vi "Queue Driver LV2.vi"(0 "States":T1[](array[typedef]), 2 "Name":string, 11 "Error In":errorcluster, 13 "Operation":T2=enum."Enqueue") -> (4 "Dequeued State":T1, 15 "error out":errorcluster)   [LabVIEW 2022 SP3, in "Sample PC Template.lvlib"]
doc: "LV2 used for queue operations\nQueue used for enqueue/dequeue of States"
uses:
  Sample PC Template.lvlib
  Typedefs/Data.ctl
  Typedefs/Queue Operations.ctl
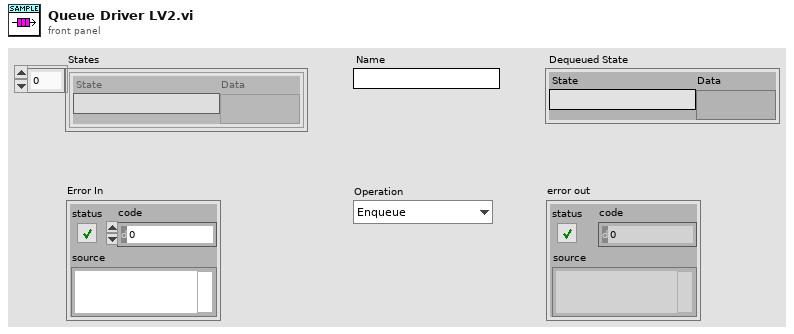
[diagram p1: front panel]
types:
  T1 = typedef "Sample PC Template.lvlib/Data.ctl" = cluster{"State":string, "Data":variant}
  T2 = typedef "Sample PC Template.lvlib/Queue Operations.ctl" = enum16{"Create Q", "Enqueue", "Enstack", "Dequeue", "Flush Q", "Release Q"}
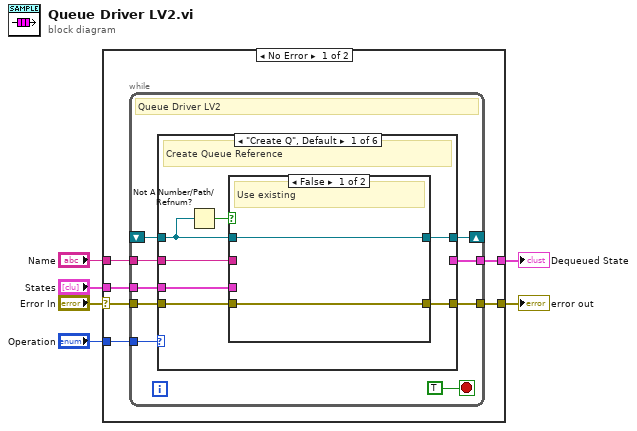
[diagram p0: block diagram]
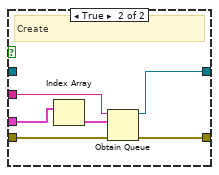
[diagram p2: hidden frame]
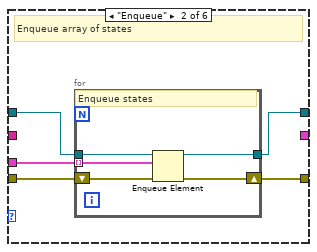
[diagram p3: hidden frame]
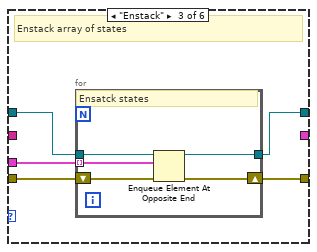
[diagram p4: hidden frame]
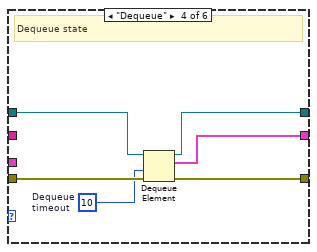
[diagram p5: hidden frame]
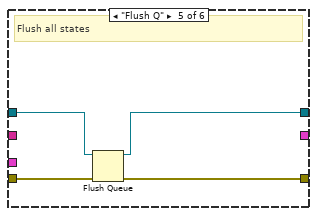
[diagram p6: hidden frame]
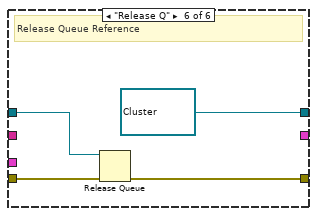
[diagram p7: hidden frame]
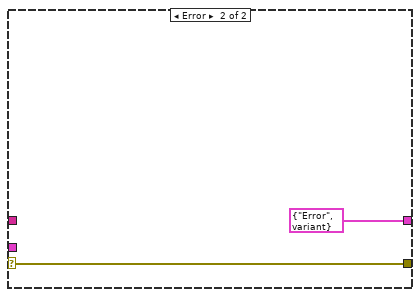
[diagram p8: hidden frame]
diagram:
  n1 = case shown="No Error" "Error In" {
    selector: "Error In" -> [w11 w72]
    tunnel: [w12 w72] -> w5
    tunnel: "Operation" -> [w10 _]
    tunnel: "Name" -> [w9 _]
    tunnel: "States" -> [w8 _]
    tunnel: [w7 T1 {"State"="Error", "Data"=variant} ("Cluster")] -> w1
    frame No Error {
      n2 = while {
        tunnel: [w21] -> w12
        tunnel: w11 -> [w20]
        tunnel: w10 -> [w19]
        tunnel: w9 -> [w16]
        tunnel: w8 -> [w15]
        shift-right: [w17] -> _
        shift-left: _ -> [w18]
        tunnel: [w14] -> w7
        stop <- TRUE stop-if-true
        # "Queue Driver LV2"
        n3 = case shown="\"Create Q\", Default" w19 {
          tunnel: [w27 w41 w51 w62 w66 w70] -> w21
          tunnel: w20 -> [w28 w40 w50 w61 w65 w69]
          tunnel: w18 -> [w22 w39 w49 w60 w64 w68]
          tunnel: [w25 w38 w48 w59 w63 refnum<queue> refnum ("queue out")] -> w17
          tunnel: w16 -> [w26 _ _ _ _ _]
          tunnel: w15 -> [w24 w37 w47 _ _ _]
          tunnel: [_ _ _ w58 _ _] -> w14
          frame "Create Q", Default {
            # "Create Queue Reference"
            n4 = Not A Number/Path/Refnum?(number/path/refnum=w22) -> (NaN/Path/Refnum?=w23:bool)
            n5 = case shown="False" w23 {
              tunnel: w28 -> [w29 w36]
              tunnel: [w29 w35] -> w27
              tunnel: w26 -> [_ w34]
              tunnel: [w30 w33] -> w25
              tunnel: w24 -> [_ w32]
              tunnel: w22 -> [w30 _]
              frame False {
                # "Use existing"
              }
              frame True {
                # "Create"
                n6 = Index Array(array=w32) -> (element=w31:T1)  [unwired: 1 in]
                n7 = Obtain Queue(name (unnamed)=w34, element data type=w31, error in (no error)=w36) -> (queue out=w33:refnum<queue>, error out=w35:errorcluster)  [unwired: 2 in, 1 out]
              }
            }
          }
          frame "Enqueue" {
            # "Enqueue array of states"
            n8 = for {
              tunnel: w39 -> [w44]
              tunnel: [w43] -> w38
              tunnel: w37 -> [w42] mode=indexing
              shift-right: [w46] -> w41
              shift-left: w40 -> [w45]
              # "Enqueue states"
              n9 = Enqueue Element(queue=w44, element=w42, error in (no error)=w45) -> (queue out=w43:refnum<queue>, error out=w46:errorcluster)  [unwired: 1 in, 1 out]
            }
          }
          frame "Enstack" {
            # "Enstack array of states"
            n10 = for {
              tunnel: w49 -> [w54]
              tunnel: [w53] -> w48
              tunnel: w47 -> [w52] mode=indexing
              shift-right: [w56] -> w51
              shift-left: w50 -> [w55]
              # "Ensatck states"
              n11 = Enqueue Element At Opposite End(queue=w54, element=w52, error in (no error)=w55) -> (queue out=w53:refnum<queue>, error out=w56:errorcluster)  [unwired: 1 in, 1 out]
            }
          }
          frame "Dequeue" {
            w57 = 10  # Dequeue timeout
            # "Dequeue state"
            n12 = Dequeue Element(queue=w60, timeout in ms (-1)=w57, error in (no error)=w61) -> (queue out=w59:refnum<queue>, element=w58:T1, error out=w62:errorcluster)  [unwired: 1 out]
          }
          frame "Flush Q" {
            # "Flush all states"
            n13 = Flush Queue(queue=w64, error in (no error)=w65) -> (queue out=w63:refnum<queue>, error out=w66:errorcluster)  [unwired: 1 out]
          }
          frame "Release Q" {
            # "Release Queue Reference"
            n14 = Release Queue(queue=w68, error in (no error)=w69) -> (error out=w70:errorcluster)  [unwired: 1 in, 2 out]
          }
        }
      }
    }
    frame Error {
    }
  }
  "error out" <- w5
  "Dequeued State" <- w1
